vi "UIRef.vi"(8 "error in":errorcluster, 11 "Engine in":refnum<class "CVT Engine Editor.lvclass">) -> (0 "error out":errorcluster, 2 "VI refnum":refnum<vi>, 3 "Engine out":refnum<class "CVT Engine Editor.lvclass">)   [LabVIEW 2013, in "CVT Engine Editor.lvclass"]
doc: "Stores the static reference to the UI of the node."
uses:
  CVT Engine Editor.lvclass
  CVTEngineUI.vi
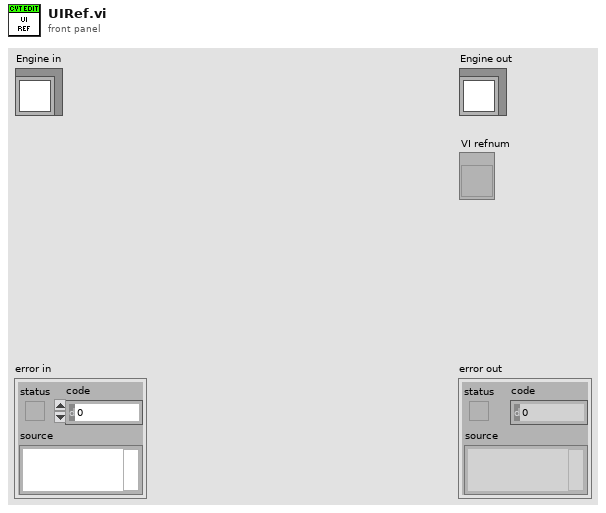
[diagram p1: front panel]
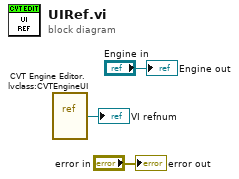
[diagram p0: block diagram]
diagram:
  n1 = vi-ref "CVT Engine Editor.lvclass:CVTEngineUI.vi"() -> (→"VI refnum":refnum<vi>)
  "error out" <- "error in"
  "Engine out" <- "Engine in"
